vi "Stamp communication 3.vi"(8 "error in (no error)":errorcluster, 10 "command array":string[](array[string]), 11 "Serial Port":refnum<visa-resource-name>) -> (0 "error out":errorcluster, 1 "Success":bool, 2 "responses":string[](array[string]), 3 "Serial Port out":refnum<visa-resource-name>, 4 "tries":i32, 6 "version":string)   [LabVIEW 2010]
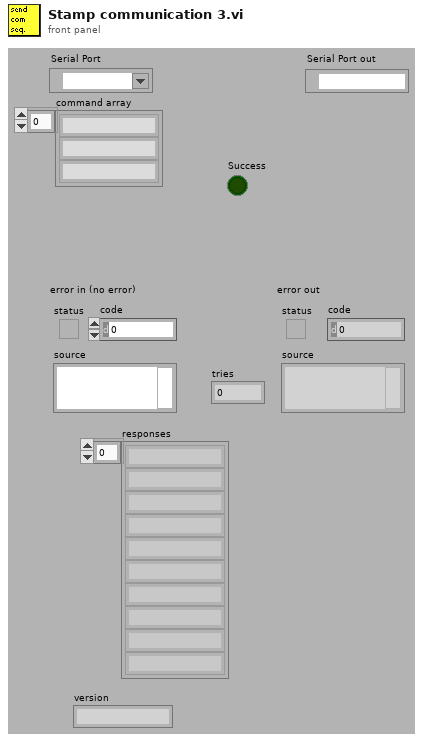
[diagram p1: front panel]
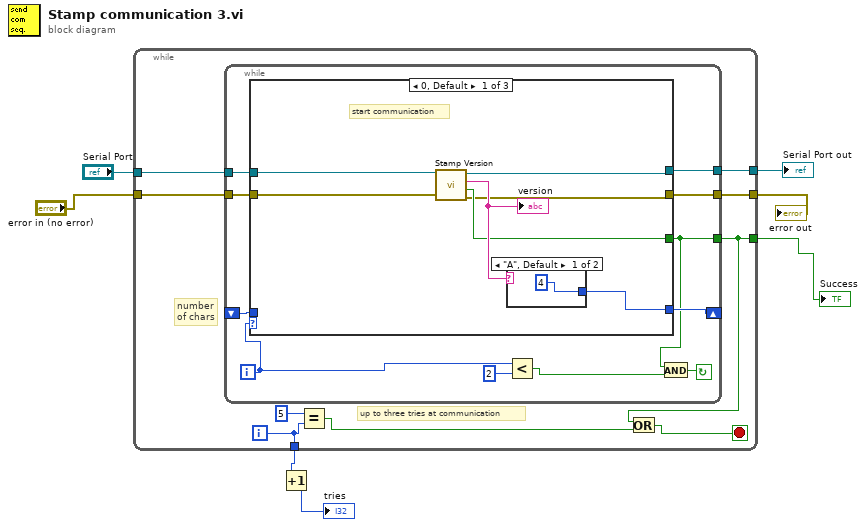
[diagram p0: block diagram]
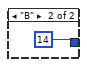
[diagram p2: hidden frame]
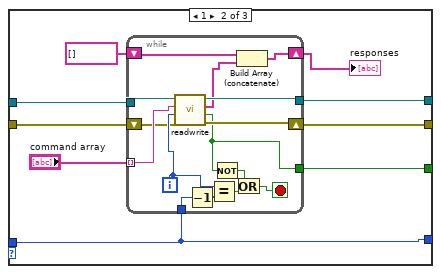
[diagram p3: hidden frame]
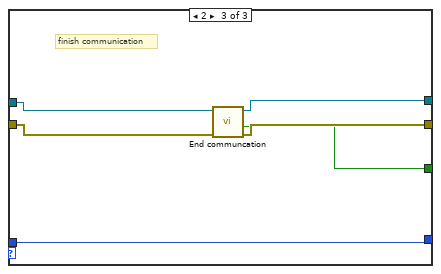
[diagram p4: hidden frame]
diagram:
  n1 = while {
    tunnel: "Serial Port" -> [w16]
    tunnel: [w15] -> w6
    tunnel: "error in (no error)" -> [w14]
    tunnel: [w13] -> w4
    tunnel: [w11] -> w3
    tunnel: [w8] -> w2
    i -> [w8]
    stop <- w12 stop-if-true
    # "number\nof chars"
    # "up to three tries at communication"
    n2 = while {
      tunnel: w16 -> [w27]
      tunnel: [w26] -> w15
      tunnel: w14 -> [w25]
      tunnel: [w24] -> w13
      tunnel: [w20] -> w11
      shift-right: [w23] -> _
      shift-left: _ -> [w22]
      i -> [w21]
      stop <- w19 continue-if-true
      n3 = case shown="0, Default" w21 {
        tunnel: w27 -> [w34 w45 w65]
        tunnel: [w33 w44 w64] -> w26
        tunnel: w25 -> [w30 w43 w63]
        tunnel: [w28 w42 w62] -> w24
        tunnel: [w29 w37 w61] -> w20
        tunnel: [w31 w40 w66] -> w23
        tunnel: w22 -> [_ w40 w66]
        frame 0, Default {
          # "start communication"
          n4 = call "Stamp Version.vi"("error in (no error)"=w30, "Serial port"=w34) -> ("error out"=w28:errorcluster, "success"=w29:bool, "version"=w32:string, "Serial port out"=w33:refnum<visa-resource-name>)  [unwired: 6 in]
          "version" <- w32
          n5 = case shown="\"A\", Default" w32 {
            tunnel: [4 14] -> w31
            frame "A", Default {
            }
            frame "B" {
            }
          }
        }
        frame 1 {
          n6 = while {
            tunnel: w45 -> [w60]
            tunnel: [w59] -> w44
            shift-right: [w51] -> w42
            shift-left: w43 -> [w52]
            tunnel: "command array" -> [w54] mode=indexing
            tunnel: w40 -> [w58]
            shift-right: [w48] -> w39
            shift-left: string[] [] -> [w47]
            tunnel: [w46] -> w37
            i -> [w53]
            stop <- w55 stop-if-true
            n7 = call "readwrite.vi"("error in (no error)"=w52, "Command ID"=w53, "Command"=w54, "Serial port"=w60) -> ("error out"=w51:errorcluster, "success"=w46:bool, "responses"=w49:string[], "Serial port out"=w59:refnum<visa-resource-name>)  [unwired: 4 in]
            n8 = Decrement(x=w58) -> (x-1=w50:i32)
            n9 = Equal?(x=w53, y=w50) -> (x = y?=w56:bool)
            n10 = Not(x=w46) -> (.not. x?=w57:bool)
            n11 = Or(x=w57, y=w56) -> (x .or. y?=w55:bool)
            n12 = Build Array (concatenate)(w47, w49) -> (w48:string[])
          }
          "responses" <- w39
        }
        frame 2 {
          # "finish communication"
          n13 = call "End communcation.vi"("error in (no error)"=w63, "Serial port"=w65) -> ("error out"=w62:errorcluster, "success"=w61:bool, "Serial port out"=w64:refnum<visa-resource-name>)  [unwired: 7 in]
        }
      }
      n14 = Less?(x=w21, y=2) -> (x < y?=w18:bool)
      n15 = And(x=w20, y=w18) -> (x .and. y?=w19:bool)
    }
    n16 = Equal?(x=5, y=w8) -> (x = y?=w10:bool)
    n17 = Or(x=w11, y=w10) -> (x .or. y?=w12:bool)
  }
  "Serial Port out" <- w6
  "error out" <- w4
  "Success" <- w3
  n18 = Increment(x=w2) -> (x+1=→"tries":i32)
